vi "Generator.Create AO DC waveforms.vi"(8 "error in (no error)":errorcluster, 9 "sweep index":i32=-1, 11 "Instrument.DAQ in":refnum<class "Instrument.DAQ.lvclass">) -> (0 "error out":errorcluster, 2 "AO Array":waveform(dbl)[](array[waveform]), 3 "Instrument.DAQ out":refnum<class "Instrument.DAQ.lvclass">)   [LabVIEW 2019, in "Instrument.DAQ.lvclass"]
uses:
  Instrument.DAQ.lvclass
panel:
  in  "Update graphs?":bool
  out "Waveform Graph":waveform(dbl)[](graph)
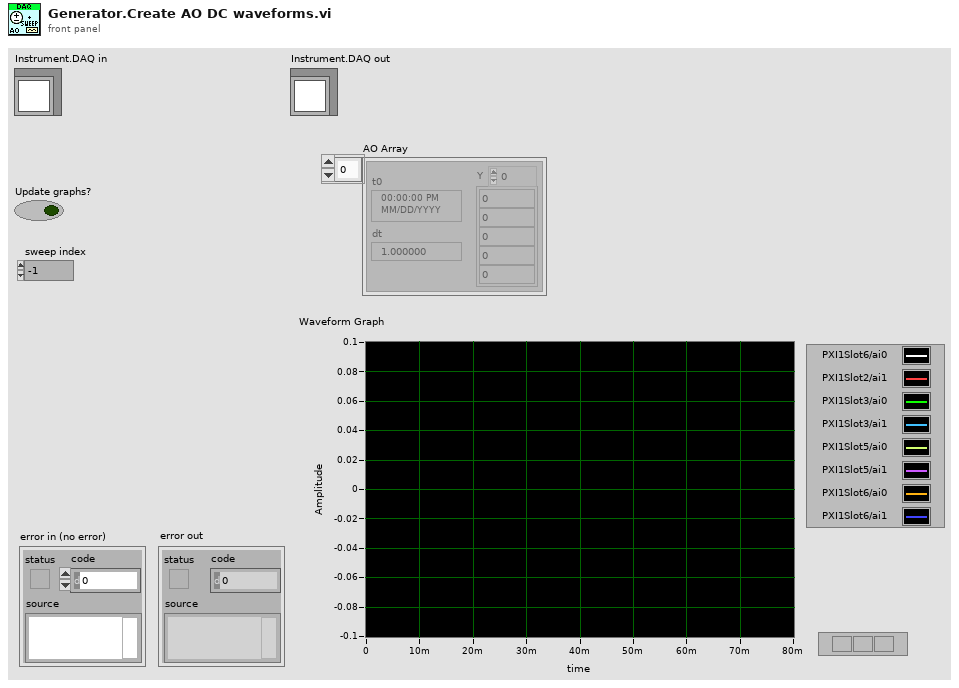
[diagram p1: front panel]
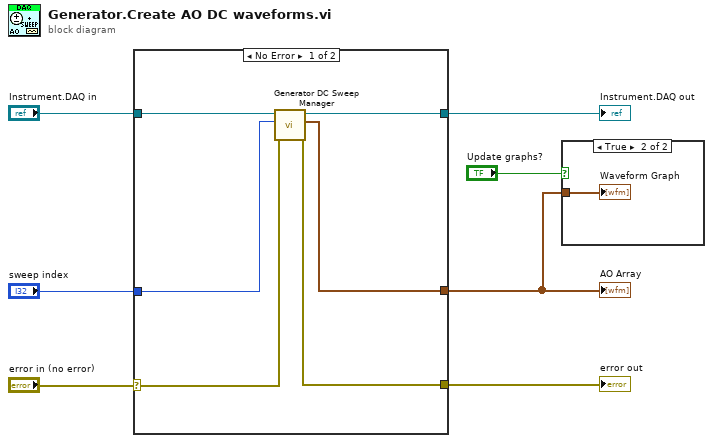
[diagram p0: block diagram]
diagram:
  n1 = case shown="No Error" "error in (no error)" {
    selector: "error in (no error)" -> [w8 w15]
    tunnel: "sweep index" -> [w13 _]
    tunnel: "Instrument.DAQ in" -> [w12 w14]
    tunnel: [w11 w14] -> w4
    tunnel: [w10 w15] -> w3
    tunnel: [w9 _] -> w2
    frame No Error {
      n2 = call "Generator DC Sweep Manager.vi"("error in (no error)"=w8, "sweep index"=w13, "Instrument.DAQ in"=w12) -> ("error out"=w10:errorcluster, "Waveform []"=w9:waveform(dbl)[], "Instrument.DAQ out"=w11:refnum<class "Instrument.DAQ.lvclass">)  [unwired: 6 in]
    }
    frame Error {
    }
  }
  "AO Array" <- w2
  "error out" <- w3
  "Instrument.DAQ out" <- w4
  n3 = case shown="True" "Update graphs?" {
    tunnel: w2 -> [_ w16]
    frame False {
    }
    frame True {
      "Waveform Graph" <- w16
    }
  }
